vi "DFConfig DFSE.vi"(8 "error in (no error)":errorcluster, 10 "DF Name":string, 11 "Desktop.DDD In":string) -> (0 "error out":errorcluster, 3 "Desktop.DDD Out":string)   [LabVIEW 2011]
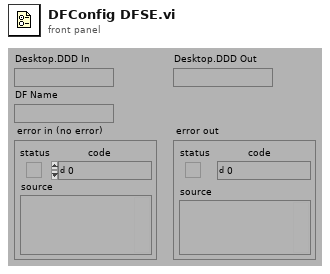
[diagram p1: front panel]
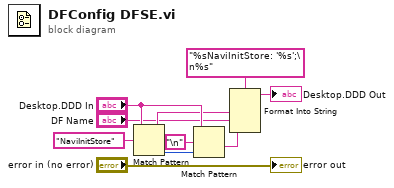
[diagram p0: block diagram]
diagram:
  n1 = Match Pattern(string="Desktop.DDD In", regular expression="NaviInitStore") -> (before substring=w6:string, offset past match=w8:i32)  [unwired: 1 in, 2 out]
  n2 = Match Pattern(string="Desktop.DDD In", regular expression="\n", offset (0)=w8) -> (after substring=w5:string)  [unwired: 3 out]
  n3 = Format Into String(format string="%sNaviInitStore: '%s';\n%s" ("regular expression"), w6, "DF Name", w5) -> (resulting string=→"Desktop.DDD Out":string)  [unwired: 2 in, 1 out]
  "error out" <- "error in (no error)"
